vi "Create Resolution.vi"(6 "행의 개수":u32, 7 "Table Ref":refnum<vi>, 8 "에러 입력(에러 없음)":errorcluster, 9 "Resolution":string[][](array[string]), 11 "Func_ext":string) -> (0 "에러 출력":errorcluster, 1 "Resolution Out":string[][](array[string]), 3 "Func_ext 출력":string)   [LabVIEW 2020]
uses:
  Controls/Cmd_Var Data IO.ctl
  Public/Polymorph/Table Initialize_2D.vi
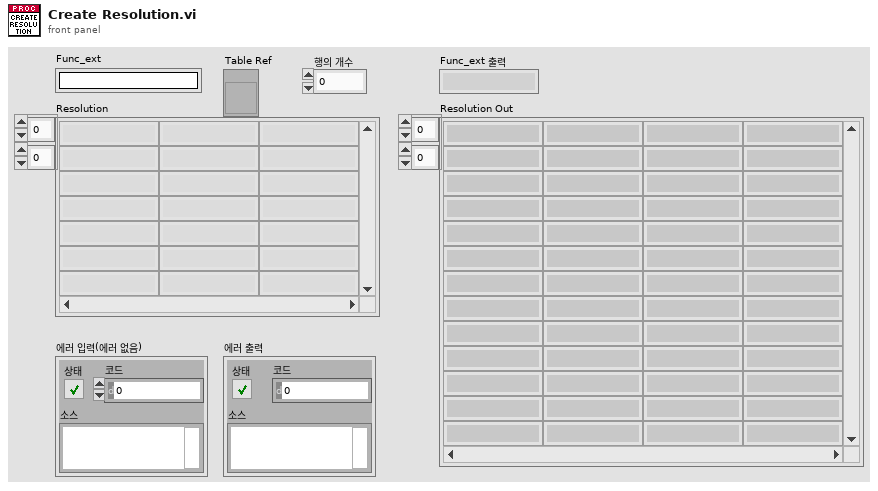
[diagram p1: front panel]
types:
  T1 = typedef "Cmd_Var Data IO.ctl" = enum16{"Condition", "Condition Default", "Condition_Temp", "Resolution", "Resolution Default", "Resolution Old", "Spec", "Spec Default", "Spec Old", "Spec Temp", "Result", "Result2", "Result3", "Result_Temp", "Result_ADJ", "Result_ADJ2", "STD1", "STD2", "STD3", "STD4", "STD5", "STD Temp", "CMC", "CMC Default"}
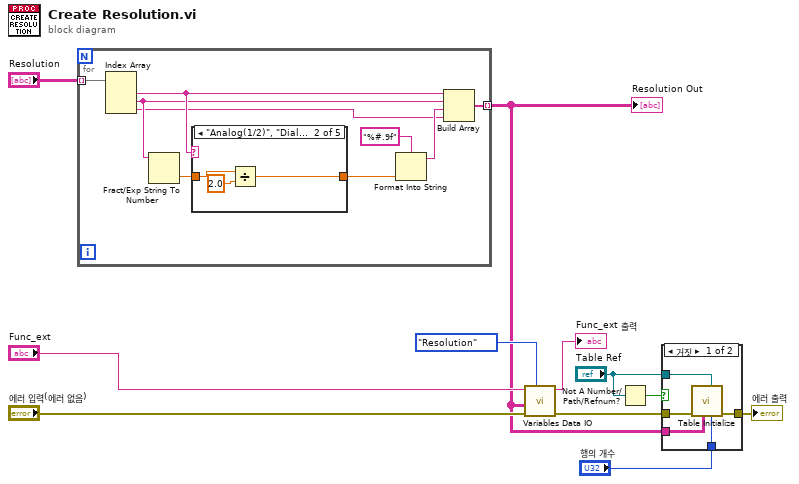
[diagram p0: block diagram]
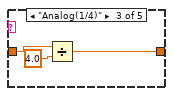
[diagram p4: hidden frame]
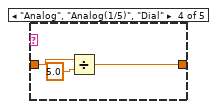
[diagram p5: hidden frame]
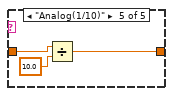
[diagram p6: hidden frame]
diagram:
  n1 = for {
    tunnel: "Resolution" -> [w17] mode=indexing
    tunnel: [w12] -> w4 mode=indexing
    n2 = Index Array(array=w17) -> (element #1=w16:string, element #2=w15:string, element #3=w13:string)  [unwired: 3 in]
    n3 = Fract/Exp String To Number(string=w15) -> (number=w20:dbl)  [unwired: 3 in, 1 out]
    n4 = case shown="\"Analog(1/2)\", \"Dial(1/2)\"" w16 {
      tunnel: w20 -> [w21 w24 w27 w30 w33]
      tunnel: [w21 w22 w25 w28 w31] -> w19
      frame "Analog(1/1)", "Digital", "Vernier", Default {
      }
      frame "Analog(1/2)", "Dial(1/2)" {
        n5 = Divide(x=w24, y=2.0) -> (x/y=w22:dbl)
      }
      frame "Analog(1/4)" {
        n6 = Divide(x=w27, y=4.0) -> (x/y=w25:dbl)
      }
      frame "Analog", "Analog(1/5)", "Dial" {
        n7 = Divide(x=w30, y=5.0) -> (x/y=w28:dbl)
      }
      frame "Analog(1/10)" {
        n8 = Divide(x=w33, y=10.0) -> (x/y=w31:dbl)
      }
    }
    n9 = Format Into String(format string="%#.9f" ("포맷 문자열"), w19) -> (resulting string=w14:string)  [unwired: 2 in, 1 out]
    n10 = Build Array(w16, w15, w14, w13) -> (w12:string[])
  }
  "Resolution Out" <- w4
  n11 = call "Variables Data IO.vi"("Select"=Cmd_Var_Data_IO."Resolution", "error in"="에러 입력(에러 없음)", "Data In"=w4, "Func_ext"="Func_ext") -> ("error out"=w6:errorcluster, "Func_ext Out"=→"Func_ext 출력":string)  [unwired: 5 in, 1 out]
  n12 = Not A Number/Path/Refnum?(number/path/refnum="Table Ref") -> (NaN/Path/Refnum?=w2:bool)
  n13 = case shown="거짓" w2 {
    tunnel: w6 -> [w38 w39]
    tunnel: [w37 w39] -> w5
    tunnel: "Table Ref" -> [w36 _]
    tunnel: w4 -> [w34 _]
    tunnel: "행의 개수" -> [w35 _]
    frame False {
      n14 = call-poly "Table Initialize.vi"("행의 개수"=w35, "Table Ref"=w36, "Value"=w34, "에러 입력"=w38) -> ("에러 출력"=w37:errorcluster)  [unwired: 5 in, 2 out]
    }
    frame True {
    }
  }
  "에러 출력" <- w5
